vi "OutControlRefnums.vi"(2 "stop":bool) -> (0 "Output Cluster":T1 {"Numeric New Value" format="%.2f"})   [LabVIEW 2013]
panel:
  in  "String Control To Change":string
  in  "Numeric Control To Change":dbl format="%0.2f"
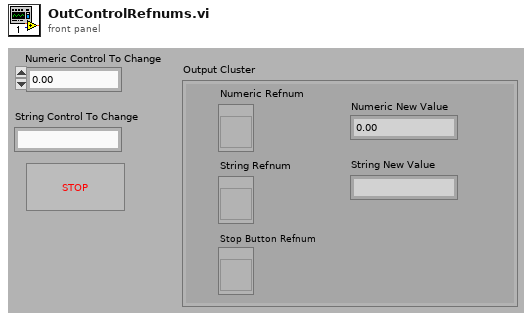
[diagram p1: front panel]
types:
  T1 = cluster{"Numeric Refnum":refnum<vi>, "String Refnum":refnum<vi>, "Stop Button Refnum":refnum<vi>, "Numeric New Value":dbl, "String New Value":string}
  T2 = cluster{"Numeric Control To Change":refnum<vi>, "String Control To Change":refnum<vi>, "stop":refnum<vi>, "Numeric Control To Change":dbl, "String Control To Change":string}
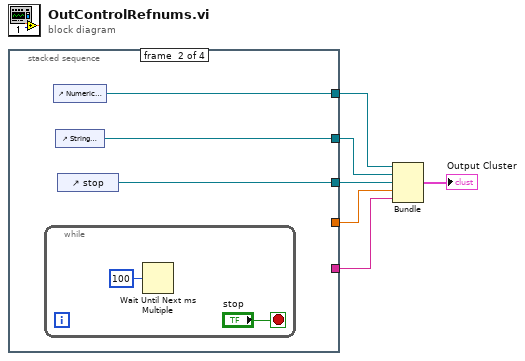
[diagram p0: block diagram]
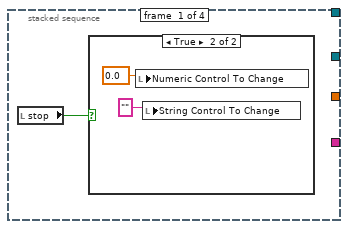
[diagram p2: hidden frame]
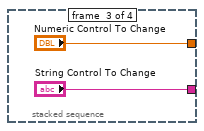
[diagram p4: hidden frame]
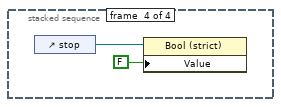
[diagram p5: hidden frame]
diagram:
  n1 = stacked-sequence {
    tunnel: [_ _ "Numeric Control To Change" _] -> w3
    tunnel: [_ _ "String Control To Change" _] -> w4
    tunnel: [_ w12 _ _] -> w6
    tunnel: [_ w11 _ _] -> w5
    tunnel: [_ w10 _ _] -> w2
    frame #0 {
      n2 = local read "stop"() -> (w7:bool)
      n3 = case shown="True" w7 {
        frame False {
        }
        frame True {
          n4 = local write "Numeric Control To Change"(0.0 ("Numeric Control To Change")) -> ()
          n5 = local write "String Control To Change"("" ("String Control To Change")) -> ()
        }
      }
    }
    frame #1 {
      n6 = while {
        stop <- "stop" stop-if-true
        n7 = Wait Until Next ms Multiple(millisecond multiple=u32 100) -> ()  [unwired: 1 out]
      }
      n8 = control-ref of="Numeric Control To Change"() -> (w12:refnum<vi>)
      n9 = control-ref of="String Control To Change"() -> (w11:refnum<vi>)
      n10 = control-ref of="stop"() -> (w10:refnum<vi>)
    }
    frame #2 {
    }
    frame #3 {
      n11 = control-ref of="stop"() -> (w17:refnum<vi>)
      n12 = property class="Bool (strict)"(reference=w17, "Value"=FALSE) -> ()  [unwired: 1 in, 2 out]
    }
  }
  n13 = Bundle("Numeric Control To Change"=w6, "String Control To Change"=w5, "stop"=w2, "Numeric Control To Change"=w3, "String Control To Change"=w4) -> (→"Output Cluster":T2)  [unwired: 1 out]
